vi "Divide Data in separe sttrings.vi"(11 "Data":string) -> (1 "ADC":i32, 2 "Temperatura":string, 3 "Humedad":string)   [LabVIEW 2019, in "Analisis.lvlib"]
doc: "In this SubVI data received is a string that will be separated in three subsections humidity,temperature and adc."
uses:
  Analisis.lvlib
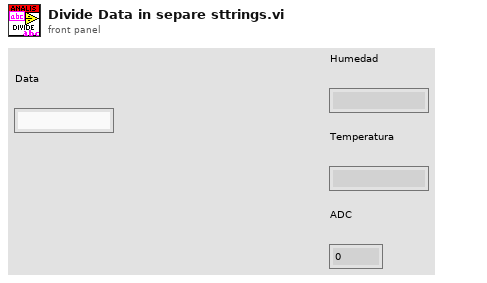
[diagram p1: front panel]
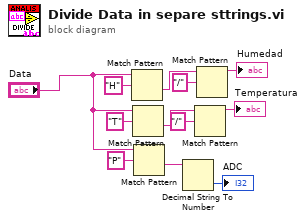
[diagram p0: block diagram]
diagram:
  n1 = Match Pattern(string="Data", regular expression="H") -> (after substring=w4:string)  [unwired: 1 in, 3 out]
  n2 = Match Pattern(string="Data", regular expression="T") -> (after substring=w7:string)  [unwired: 1 in, 3 out]
  n3 = Match Pattern(string="Data", regular expression="P") -> (after substring=w11:string)  [unwired: 1 in, 3 out]
  n4 = Decimal String To Number(string=w11) -> (number=→"ADC":i32)  [unwired: 2 in, 1 out]
  n5 = Match Pattern(string=w7, regular expression="/") -> (before substring=→"Temperatura":string)  [unwired: 1 in, 3 out]
  n6 = Match Pattern(string=w4, regular expression="/") -> (before substring=→"Humedad":string)  [unwired: 1 in, 3 out]
